vi "to string array.vi"(8 "error in (no error)":errorcluster, 11 "module configuration in":refnum<class "tag select module configuration.lvclass">) -> (0 "error out":errorcluster, 1 "Array":string[][](array[string]), 2 "version":string, 3 "module configuration out":refnum<class "tag select module configuration.lvclass">)   [LabVIEW 2015, in "tag select module configuration.lvclass"]
uses:
  tag select module configuration.lvclass
  tag select module configuration.lvclass/tag select module configuration.ctl
  Read tag select.vi
  current version.vi
  <vilib>/NI/Tag Bus Module Framework/channel/TBM channel.lvclass
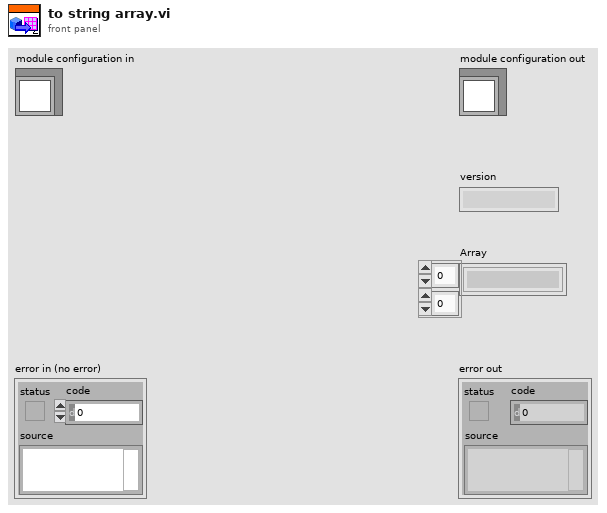
[diagram p1: front panel]
types:
  T1 = typedef "tag select module configuration.lvclass/tag select configuration.ctl" = cluster{"tag select name":string, "data type":T2, "output":refnum<class "TBM channel.lvclass">, "select":refnum<class "TBM channel.lvclass">, "input channels":refnum<class "TBM channel.lvclass">[]}
  T2 = typedef "tag bus.lvlib/tag descriptor.lvclass/Data Type.ctl" = enum16{"Double", "Single", "I64", "I32", "I16", "I8", "U64", "U32", "U16", "U8", "Boolean", "String", "Array of Double", "Array of Single", "Array of I64", "Array of I32", "Array of I16", "Array of I8", "Array of U64", "Array of U32", "Array of U16", "Array of U8", "Array of Boolean", "Array of String"}
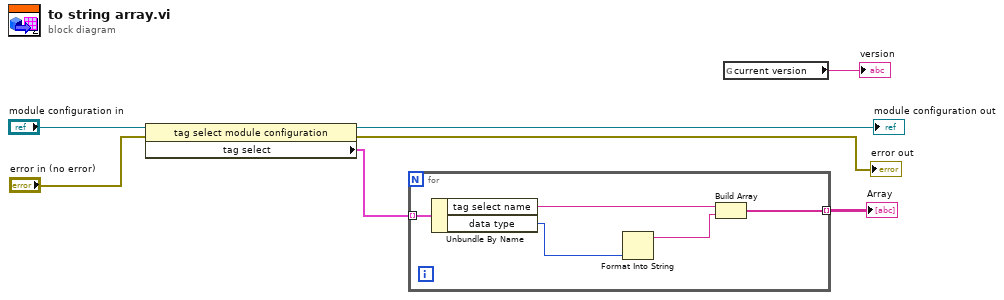
[diagram p0: block diagram]
diagram:
  n1 = property class="tag select module configuration"(reference="module configuration in", error in="error in (no error)") -> (reference out=→"module configuration out":refnum<class "tag select module configuration.lvclass">, error out=→"error out":errorcluster, "tag select"=w3:T1[])
  n2 = for {
    tunnel: w3 -> [w12] mode=indexing
    tunnel: [w8] -> w2 mode=indexing
    n3 = Unbundle By Name(w12) -> ("tag select name"=w11:string, "data type"=w10:T2)
    n4 = Format Into String(w10) -> (resulting string=w9:string)  [unwired: 3 in, 1 out]
    n5 = Build Array(w11, w9) -> (w8:string[])
  }
  "Array" <- w2
  n6 = global read "current version.vi" "current version"() -> (→"version":string)
